vi "Process_calibration.vi"() -> ()   [LabVIEW 2015]
uses:
  <vilib>/Analysis/5stat.llb/RMS (DBL).vi
  <vilib>/Analysis/NI_AALPro.lvlib
panel:
  out "Reporting 4":string
  out "CALIBRATION OK":bool
  out "Measurements OK":bool
  out "Reporting 3":string
  out "Valid\nfrequency":bool
  out "Reporting 2":string
  out "OK measurements":bool[](array[boolean])
  out "Waveform Graph 4":waveform(dbl)[](graph)
  out "Calibration\nparameter":dbl
  out "Sensivity\ncalibrated\nmV/g":dbl
  in  "Pattern\namplitude":dbl=1.02
  out "Valid\nmeasur\nfrequency":bool[](array[boolean])
  out "Reporting":string
  out "All Files in Dir":path[](array[path])
  in  "Frecuencia\nmuestreo":dbl=25600.0
  in  "Pattern frequency (Hz)":dbl=159.2
  in  "Nº canales":i32=10
  in  "Folder Path":path
  # "Min"
  # "Median"
  # "Mean"
  # "Variance"
  # "Max"
  # "G:\\Mi unidad\\WRD\\SERVICIOS_Disco_duro\\Euskotren\\Lugaritz\\2016-05\\Calibracion\\4D\\verde"
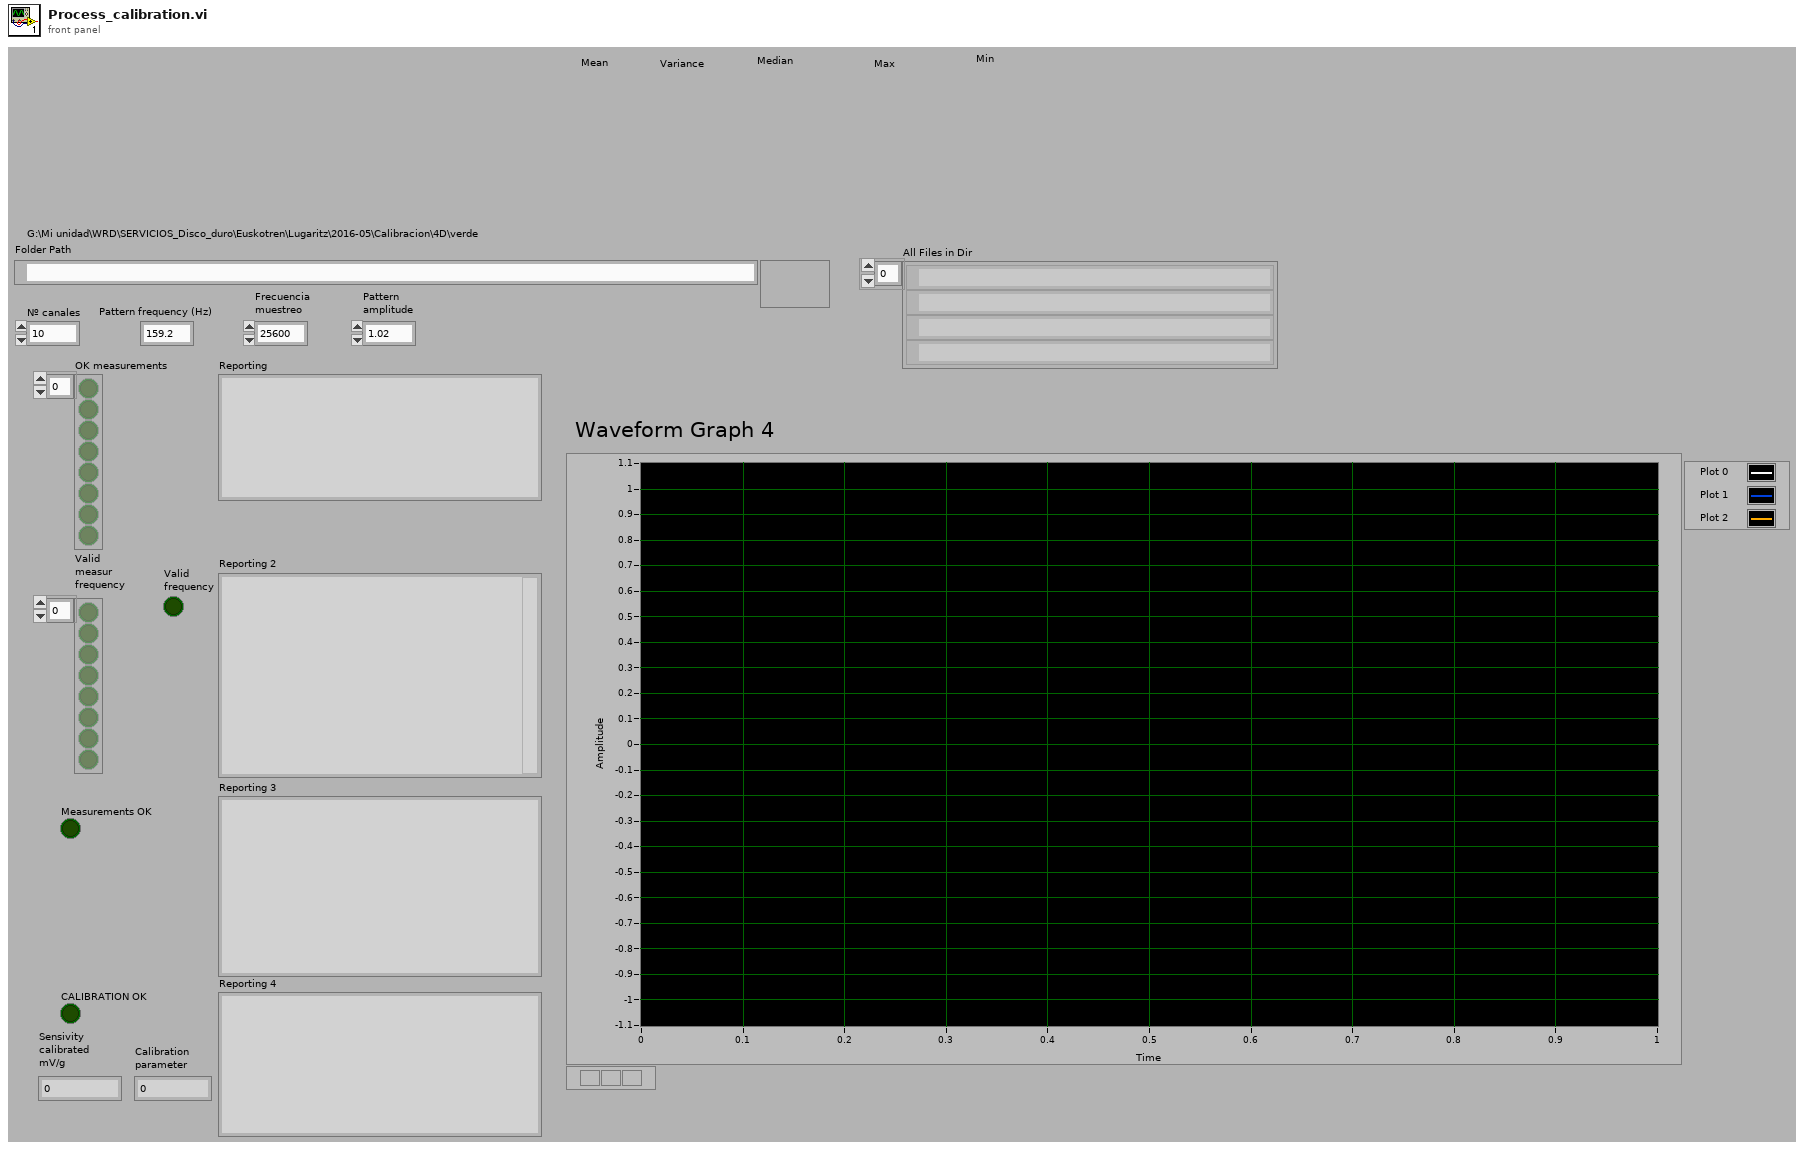
[diagram p1: front panel]
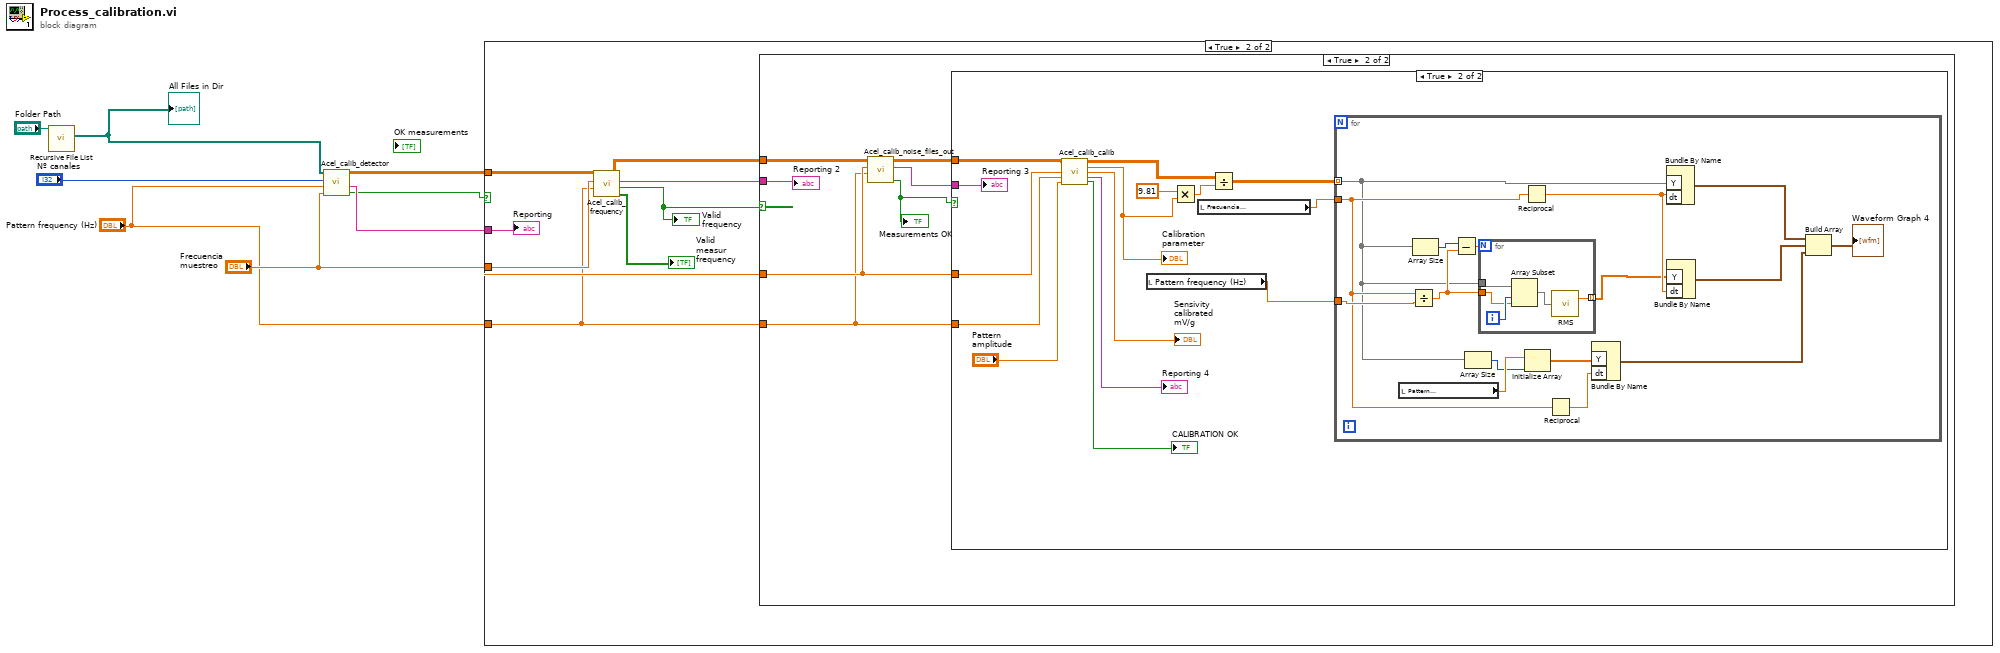
[diagram p0: block diagram]
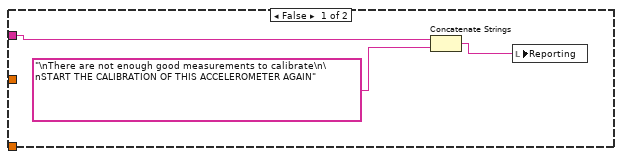
[diagram p2: hidden frame]
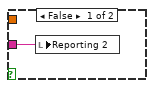
[diagram p3: hidden frame]
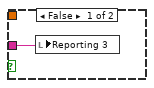
[diagram p4: hidden frame]
diagram:
  n1 = call <vilib>:"Recursive File List.vi"("Folder Path"="Folder Path") -> ("All Files in Dir"=w6:path[])  [unwired: 6 in, 4 out]
  "All Files in Dir" <- w6
  n2 = call "Acel_calib_detector.vi"("Frecuencia\nmuestreo"="Frecuencia\nmuestreo", "Pattern frequency (Hz)"="Pattern frequency (Hz)", "Nº canales"="Nº canales", "All Files in Dir"=w6) -> ("Continue calibrating?"=w1:bool, "Reporting"=w2:string, "Acel Cal measurements"=w8:sgl[][])  [unwired: 1 out]
  n3 = case shown="True" w1 {
    tunnel: w8 -> [_ w19]
    tunnel: "Frecuencia\nmuestreo" -> [_ w17]
    tunnel: "Pattern frequency (Hz)" -> [_ w16]
    tunnel: w2 -> [w11 w15]
    frame False {
      n4 = Concatenate Strings(w11, "\nThere are not enough good measurements to calibrate\n\nSTART THE CALIBRATION OF THIS ACCELEROMETER AGAIN" ("Reporting")) -> (w9:string)
      n5 = local write "Reporting"(w9) -> ()
    }
    frame True {
      n6 = call "Acel_calib_frequency.vi"("Pattern frequency (Hz)"=w16, "Frecuencia\nmuestreo"=w17, "Acel Cal measurements in"=w19) -> ("Measurements OK"=→"Valid\nmeasur\nfrequency":bool[], "Valid frequency"=w14:bool, "Reporting2"=w13:string, "Acel Cal measurements out"=w18:sgl[][])  [unwired: 1 in]
      "Valid\nfrequency" <- w14
      n7 = case shown="True" w14 {
        tunnel: w18 -> [_ w27]
        tunnel: w17 -> [_ w26]
        tunnel: w16 -> [_ w25]
        tunnel: w13 -> [w20 w22]
        frame False {
          n8 = local write "Reporting 2"(w20) -> ()
        }
        frame True {
          n9 = call "Acel_calib_noise_files_out.vi"("Pattern frequency (Hz)"=w25, "Frecuencia\nmuestreo"=w26, "Acel Cal measurements in"=w27) -> ("Measurements OK"=w21:bool, "Reporting 3"=w24:string, "Acel Cal measurements out 2"=w23:sgl[][])  [unwired: 6 in]
          "Measurements OK" <- w21
          n10 = case shown="True" w21 {
            tunnel: w26 -> [_ w43]
            tunnel: w25 -> [_ w42]
            tunnel: w24 -> [w28 w38]
            tunnel: w23 -> [_ w35]
            frame False {
              n11 = local write "Reporting 3"(w28) -> ()
            }
            frame True {
              n12 = call "Acel_calib_calib.vi"("Acel Cal measurements in"=w35, "Frecuencia\nmuestreo"=w43, "Pattern frequency (Hz)"=w42, "Pattern\namplitude"="Pattern\namplitude") -> ("Acel Cal measurements out"=w30:dbl[][], "Calibration parameter"=w29:dbl, "Sensivity (mV/g)"=→"Sensivity\ncalibrated\nmV/g":dbl, "Reporting 4"=→"Reporting 4":string, "Calibration OK"=→"CALIBRATION OK":bool)  [unwired: 7 in]
              "Calibration\nparameter" <- w29
              n13 = local read "Pattern frequency (Hz)"() -> (w40:dbl)
              n14 = Multiply(x=9.81 ("y"), y=w29) -> (x*y=w36:dbl)
              n15 = local read "Frecuencia\nmuestreo"() -> (w39:dbl)
              n16 = Divide(x=w30, y=w36) -> (x/y=w41:dbl[][])
              n17 = for {
                tunnel: w41 -> [w45] mode=indexing
                tunnel: w40 -> [w57]
                tunnel: w39 -> [w47]
                n18 = local read "Pattern\namplitude"() -> (w50:dbl)
                n19 = Divide(x=w47, y=w57) -> (x/y=w56:dbl)
                n20 = Array Size(array=w45) -> (size(s)=w58:i32)
                n21 = Subtract(x=w58, y=w56) -> (x-y=w59:dbl)
                n22 = Array Size(array=w45) -> (size(s)=w49:i32)
                n23 = for {
                  N: w59 -> [_]
                  tunnel: w56 -> [w61]
                  tunnel: [w64] -> w44 mode=indexing
                  tunnel: w45 -> [w63]
                  i -> [w62]
                  n24 = Array Subset(array=w63, index=w62, length=w61) -> (w60:dbl[])
                  n25 = call-poly <vilib>:"RMS.vi"("X"=w60) -> ("rms value"=w64:dbl)  [unwired: 1 out]
                }
                n26 = Reciprocal(x=w47) -> (1/x=w55:dbl)
                n27 = Initialize Array(w50, w49) -> (w48:dbl[])
                n28 = Reciprocal(x=w47) -> (1/x=w51:dbl)
                n29 = Bundle By Name("Y"=w48, "dt"=w51) -> (w46:waveform(dbl))  [unwired: 1 in]
                n30 = Bundle By Name("Y"=w45, "dt"=w55) -> (w53:waveform(dbl))  [unwired: 1 in]
                n31 = Bundle By Name("Y"=w44, "dt"=w55) -> (w52:waveform(dbl))  [unwired: 1 in]
                n32 = Build Array(w53, w52, w46) -> (→"Waveform Graph 4":waveform(dbl)[])
              }
              "Reporting 3" <- w38
            }
          }
          "Reporting 2" <- w22
        }
      }
      "Reporting" <- w15
    }
  }
